vi "RWA Write Strings to File.vi"(8 "Error In":errorcluster, 9 "Section Name":string, 10 "Strings[]":string[](array[string]), 11 "Path":path) -> (0 "Error Out":errorcluster, 2 "Section Replaced?":bool)   [LabVIEW 2020]
doc: "This VI was created for use with the Read/Write Cluster VIs. It writes the cluster element strings to the specified section in an INI file without editing any other sections.\n\nAuthored by Robert C. Mortensen\nsupport@mooregoodideas.com\nwww.mooregoodideas.com\n\nCopyright (c) 2010, Moore Good Ideas, Inc.\n\nAll rights reserved.\n\nRedistribution and use in source and binary forms, with or without modification, are permitted provided that the following conditions are met:\n\n * Redistributions of source code must retain the above copyright notice, this list of conditions and the following disclaimer.\n * Redistributions in binary form must reproduce the above copyright notice, this list of conditions and the following disclaimer in the documentation and/or other materials provided with the distribution.\n * Neither the name of Moore Good Ideas, Inc. nor the names of its contributors may be used to endorse or promote products derived from this software without specific prior written permission.\n\nTHIS SOFTWARE IS PROVIDED BY THE COPYRIGHT HOLDERS AND CONTRIBUTORS \"AS IS\" AND ANY EXPRESS OR IMPLIED WARRANTIES, INCLUDING, BUT NOT LIMITED TO, THE IMPLIED WARRANTIES OF MERCHANTABILITY AND FITNESS FOR A PARTICULAR PURPOSE ARE DISCLAIMED. IN NO EVENT SHALL THE COPYRIGHT OWNER OR CONTRIBUTORS BE LIABLE FOR ANY DIRECT, INDIRECT, INCIDENTAL, SPECIAL, EXEMPLARY, OR CONSEQUENTIAL DAMAGES (INCLUDING, BUT NOT LIMITED TO, PROCUREMENT OF SUBSTITUTE GOODS OR SERVICES; LOSS OF USE, DATA, OR PROFITS; OR BUSINESS INTERRUPTION) HOWEVER CAUSED AND ON ANY THEORY OF LIABILITY, WHETHER IN CONTRACT, STRICT LIABILITY, OR TORT (INCLUDING NEGLIGENCE OR OTHERWISE) ARISING IN ANY WAY OUT OF THE USE OF THIS SOFTWARE, EVEN IF ADVISED OF THE POSSIBILITY OF SUCH DAMAGE."
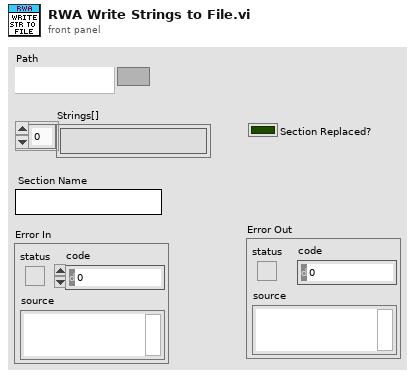
[diagram p1: front panel]
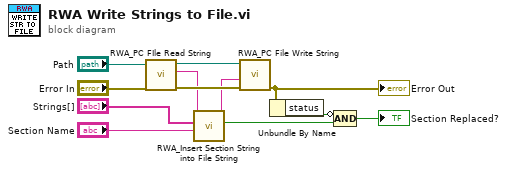
[diagram p0: block diagram]
diagram:
  n1 = call "RWA_PC FIle Read String.vi"("Error"="Error In", "Path"="Path") -> ("Error Out"=w9:errorcluster, "String Out"=w8:string, "Duplicate Path Out"=w11:path)  [unwired: 6 in, 1 out]
  n2 = call "RWA_Insert Section String into File String.vi"("Section Name"="Section Name", "Strings[]"="Strings[]", "File String"=w8) -> ("Section Replaced Out"=w5:bool, "File String Out"=w3:string)  [unwired: 7 in]
  n3 = call "RWA_PC File Write String.vi"("Error"=w9, "String"=w3, "Path"=w11) -> ("Error Out"=w7:errorcluster)  [unwired: 7 in, 1 out]
  "Error Out" <- w7
  n4 = Unbundle By Name(w7) -> ("status"=w6:bool)
  n5 = Compound Arithmetic op=AND(invert w6, w5) -> (→"Section Replaced?":bool)
